vi "Display Message.vi"(6 "Enable Lower Message (T: Enable)":bool=TRUE, 7 "Enable Upper Message (T: Enable)":bool=TRUE, 8 "error in (no error)":errorcluster, 9 "Lower Message (\"Message\")":string="Message", 10 "Upper Message (\"Default\")":string="Default", 11 "VISA resource name":refnum<visa-resource-name>) -> (0 "error out":errorcluster, 3 "VISA resource name out":refnum<visa-resource-name>)   [LabVIEW 2020, in "Keithley 2450.lvlib"]
doc: "Displays a message on the instrument's User display."
uses:
  <instrlib>/Keithley 2450/Keithley 2450.lvlib
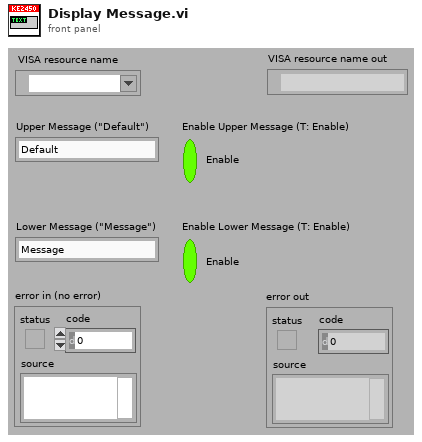
[diagram p1: front panel]
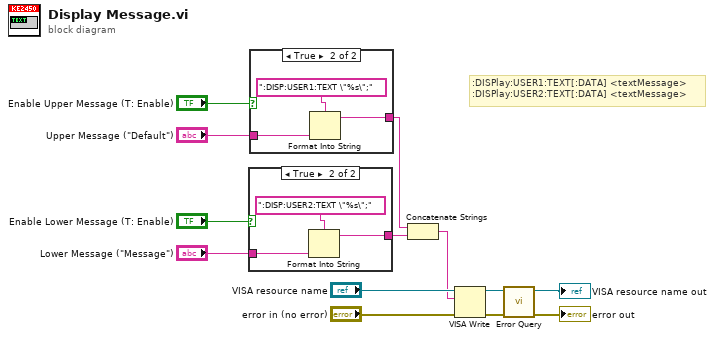
[diagram p0: block diagram]
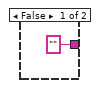
[diagram p2: hidden frame]
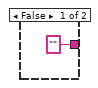
[diagram p3: hidden frame]
diagram:
  # ":DISPlay:USER1:TEXT[:DATA] <textMessage>\n:DISPlay:USER2:TEXT[:DATA] <textMessage>"
  n1 = case shown="True" "Enable Lower Message (T: Enable)" {
    tunnel: ["" w17] -> w1
    tunnel: "Lower Message (\"Message\")" -> [_ w15]
    frame False {
    }
    frame True {
      n2 = Format Into String(format string=":DISP:USER2:TEXT \"%s\";", w15) -> (resulting string=w17:string)  [unwired: 2 in, 1 out]
    }
  }
  n3 = case shown="True" "Enable Upper Message (T: Enable)" {
    tunnel: ["" w21] -> w7
    tunnel: "Upper Message (\"Default\")" -> [_ w19]
    frame False {
    }
    frame True {
      n4 = Format Into String(format string=":DISP:USER1:TEXT \"%s\";", w19) -> (resulting string=w21:string)  [unwired: 2 in, 1 out]
    }
  }
  n5 = Concatenate Strings(w7, w1) -> (w2:string)
  n6 = VISA Write(VISA resource name="VISA resource name", write buffer=w2, error in (no error)="error in (no error)") -> (VISA resource name out=w11:refnum<visa-resource-name>, error out=w8:errorcluster)  [unwired: 1 out]
  n7 = call <instrlib>:"Error Query.vi"("error in (no error)"=w8, "VISA resource name"=w11) -> ("error out"=→"error out":errorcluster, "VISA resource name out"=→"VISA resource name out":refnum<visa-resource-name>)  [unwired: 8 out]
